vi "Interpret Device Info.vi"(8 "Error In":errorcluster, 11 "Data In":u8[](array[numeric])) -> (0 "Error Out":errorcluster, 1 "Build Number":u16, 2 "Minor Version":u8, 3 "Major Version":u8, 4 "ADS Error":T1 items=["NoError"=0, "InternalError"=1, "NoRTime"=2, "LockedMemoryError"=3, "MailBoxError"=4, "WrongHMsg"=5, "TargetPortNotFound"=6, "TargetMachineNotFound"=7, "UnknownCommandID"=8, "BadTaskID"=9, "NoIO"=10, "UnknownAmsCommand"=11, "Win32Error"=12, "PortNotConnected"=13, "InvalidAmsLength"=14, "InvalidAmsNetID"=15, "AmsSyncAmsError"=22, "AmsSyncNoIndexMap"=23, "InvalidAmsPort"=24, "NoMemory"=25, "TCPSendError"=26, "HostUnreachable"=27, "NoLockedMemory"=1280, "MailboxFull"=1282, "DeviceError"=1792, "DeviceServiceNotSupported"=1793, "DeviceInvalidGroup"=1794, "DeviceInvalidOffset"=1795, "DeviceInvalidAccess"=1796, "DeviceInvalidSize"=1797, "DeviceInvalidData"=1798, "DeviceNotReady"=1799, "DeviceBusy"=1800, "DeviceInvalidContext"=1801, "DeviceNoMemory"=1802, "DeviceInvalidParam"=1803, "DeviceNotFound"=1804, "DeviceSyntaxError"=1805, "DeviceIncompatible"=1806, "DeviceExists"=1807, "DeviceSymboldNotFound"=1808, "DeviceSymbolVersionInvalid"=1809, "DeviceInvalidState"=1810, "DeviceTransModeNotSupported"=1811, "DeviceNotifyHandleInvalid"=1812, "DeviceClientUnknown"=1813, "DeviceNoMoreHandles"=1814, "DeviceInvalidWatchsize"=1815, "DeviceNotInitialized"=1816, "DeviceTimeOut"=1817, "DeviceNoInterface"=1818, "DeviceInvalidInterface"=1819, "DeviceInvalidCLSID"=1820, "DeviceInvalidObjectID"=1821, "ClientError"=1856, "ClientInvalidParameter"=1857, "ClientListEmpty"=1858, "ClientVariableInUse"=1859, "ClientDuplicateInvokeID"=1860, "ClientSyncTimeOut"=1861, "ClientW32OR"=1862, "ClientTimeoutInvalid"=1863, "ClientPortNotOpen"=1864, "ClientNoAmsAddr"=1865, "ClientSyncInternal"=1872, "ClientAddHash"=1873, "ClientRemoveHash"=1874, "ClientNoMoreSymbols"=1875, "ClientSyncResInvalid"=1876, "ClientSyncPortLocked"=1877, "ClientQueueFull"=1878], 5 "Device Name":string)   [LabVIEW 2016, in "TwinCAT ADS.lvlib"]
uses:
  TwinCAT ADS.lvlib
  TypeDefs/ADS Error.ctl
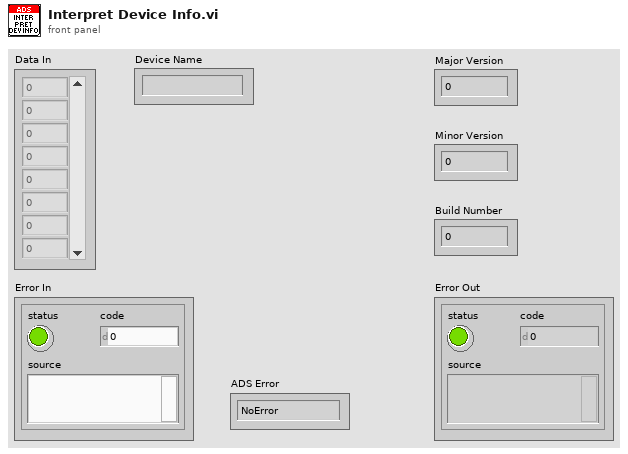
[diagram p1: front panel]
types:
  T1 = typedef "TwinCAT ADS.lvlib/ADS Error.ctl" = u32
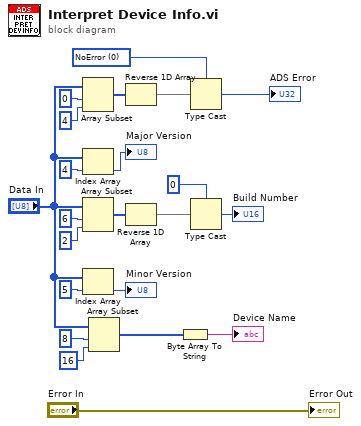
[diagram p0: block diagram]
diagram:
  w1 = T1 0 items=["NoError"=0, "InternalError"=1, "NoRTime"=2, "LockedMemoryError"=3, "MailBoxError"=4, "WrongHMsg"=5, "TargetPortNotFound"=6, "TargetMachineNotFound"=7, "UnknownCommandID"=8, "BadTaskID"=9, "NoIO"=10, "UnknownAmsCommand"=11, "Win32Error"=12, "PortNotConnected"=13, "InvalidAmsLength"=14, "InvalidAmsNetID"=15, "AmsSyncAmsError"=22, "AmsSyncNoIndexMap"=23, "InvalidAmsPort"=24, "NoMemory"=25, "TCPSendError"=26, "HostUnreachable"=27, "NoLockedMemory"=1280, "MailboxFull"=1282, "DeviceError"=1792, "DeviceServiceNotSupported"=1793, "DeviceInvalidGroup"=1794, "DeviceInvalidOffset"=1795, "DeviceInvalidAccess"=1796, "DeviceInvalidSize"=1797, "DeviceInvalidData"=1798, "DeviceNotReady"=1799, "DeviceBusy"=1800, "DeviceInvalidContext"=1801, "DeviceNoMemory"=1802, "DeviceInvalidParam"=1803, "DeviceNotFound"=1804, "DeviceSyntaxError"=1805, "DeviceIncompatible"=1806, "DeviceExists"=1807, "DeviceSymboldNotFound"=1808, "DeviceSymbolVersionInvalid"=1809, "DeviceInvalidState"=1810, "DeviceTransModeNotSupported"=1811, "DeviceNotifyHandleInvalid"=1812, "DeviceClientUnknown"=1813, "DeviceNoMoreHandles"=1814, "DeviceInvalidWatchsize"=1815, "DeviceNotInitialized"=1816, "DeviceTimeOut"=1817, "DeviceNoInterface"=1818, "DeviceInvalidInterface"=1819, "DeviceInvalidCLSID"=1820, "DeviceInvalidObjectID"=1821, "ClientError"=1856, "ClientInvalidParameter"=1857, "ClientListEmpty"=1858, "ClientVariableInUse"=1859, "ClientDuplicateInvokeID"=1860, "ClientSyncTimeOut"=1861, "ClientW32OR"=1862, "ClientTimeoutInvalid"=1863, "ClientPortNotOpen"=1864, "ClientNoAmsAddr"=1865, "ClientSyncInternal"=1872, "ClientAddHash"=1873, "ClientRemoveHash"=1874, "ClientNoMoreSymbols"=1875, "ClientSyncResInvalid"=1876, "ClientSyncPortLocked"=1877, "ClientQueueFull"=1878] ("ADS Error")
  n1 = Array Subset(array="Data In", index=0, length=4) -> (w22:u8[])
  n2 = Index Array(array="Data In", index=4) -> (element=→"Major Version":u8)
  n3 = Array Subset(array="Data In", index=6, length=2) -> (w16:u8[])
  n4 = Index Array(array="Data In", index=5) -> (element=→"Minor Version":u8)
  n5 = Array Subset(array="Data In", index=8, length=16) -> (w3:u8[])
  n6 = Reverse 1D Array(array=w22) -> (reversed array=w19:u8[])
  n7 = Reverse 1D Array(array=w16) -> (reversed array=w14:u8[])
  n8 = Byte Array To String(unsigned byte array=w3) -> (string=→"Device Name":string)
  n9 = Type Cast(type=w1, x=w19) -> (*(type *) &x=→"ADS Error":T1)
  n10 = Type Cast(type=u16 0, x=w14) -> (*(type *) &x=→"Build Number":u16)
  "Error Out" <- "Error In"
